vi "Logging Write.vi"(3 "error in (no error)":errorcluster, 5 "LoggingDevRef":T1) -> (0 "error out":errorcluster, 1 "Count":u32, 2 "LoggingDevRef":T1)   [LabVIEW 2012, in "femtoRoboLib.lvlib"]
doc: "Actually write unsaved log changes to to specified Logging reference. To prevent data loss, Flushing occasionally is recommended. Returns the number of changes written."
uses:
  femtoRoboLib.lvlib
  Controls/LoggingDevRef.ctl
  Controls/Logging Cache - Mode.ctl
  Controls/Log Entry - Written Block.ctl
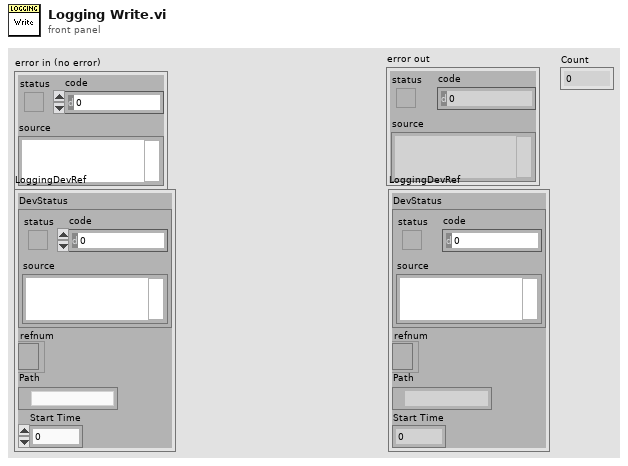
[diagram p1: front panel]
types:
  T1 = typedef "femtoRoboLib.lvlib/LoggingDevRef.ctl" = cluster{"DevStatus":errorcluster, "refnum":refnum<file>, "Path":path, "Start Time":u32}
  T2 = typedef "Log Entry - Written Block.ctl" = cluster{"ID":u32, "Value":string, "Type":enum16{"Boolean", "Numeric", "String", "Boolean Array", "Numeric Array", "String Array"}}
  T3 = typedef "Logging Cache - Mode.ctl" = enum16{"Set", "Get All", "Get Unsaved", "Get Unsaved and Clear", "Get New", "Get New and Clear"}
  T4 = typedef "femtoRoboLib.lvlib/Log Entry - Converted.ctl" = cluster{"Name":string, "Type":enum16{"Boolean", "Numeric", "String", "Boolean Array", "Numeric Array", "String Array"}, "Value":string, "ID":u32}
  T5 = enum16{"Boolean", "Numeric", "String", "Boolean Array", "Numeric Array", "String Array"}
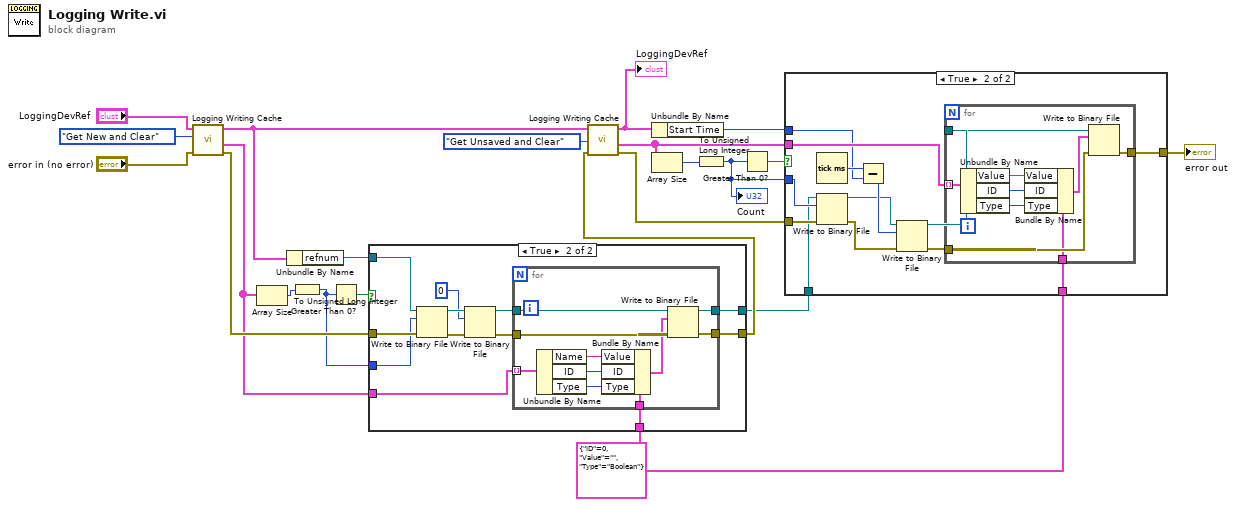
[diagram p0: block diagram]
diagram:
  w2 = T2 {"ID"=0, "Value"="", "Type"=enum."Boolean"} ("Log Entry - Written Block")
  n1 = call "Logging Writing Cache.vi"("error in (no error)"="error in (no error)", "Mode"=Logging_Cache_-_Mode."Get New and Clear", "LoggingDevRef"="LoggingDevRef") -> ("error out"=w6:errorcluster, "Out"=w4:T4[], "LoggingDevRef"=w8:T1)  [unwired: 2 in]
  n2 = Array Size(array=w4) -> (size(s)=w10:i32)
  n3 = Unbundle By Name(w8) -> ("refnum"=w7:refnum<file>)
  n4 = To Unsigned Long Integer(number=w10) -> (unsigned 32bit integer=w5:u32)
  n5 = Greater Than 0?(x=w5) -> (x > 0?=w9:bool)
  n6 = case shown="True" w9 {
    tunnel: w7 -> [w23 w36]
    tunnel: w6 -> [w24 w35]
    tunnel: w5 -> [_ w25]
    tunnel: w4 -> [_ w30]
    tunnel: [w24 w29] -> w3
    tunnel: w2 -> [_ w28]
    tunnel: [w23 w27] -> w1
    frame False {
    }
    frame True {
      n7 = Write to Binary File(file (use dialog)=w36, data=w25, error in=w35) -> (refnum out=w33:refnum<file>, error out=w34:errorcluster)  [unwired: 3 in, 1 out]
      n8 = Write to Binary File(file (use dialog)=w33, data=u32 0, error in=w34) -> (refnum out=w32:refnum<file>, error out=w31:errorcluster)  [unwired: 3 in, 1 out]
      n9 = for {
        tunnel: [w46] -> w29
        tunnel: w32 -> [w45]
        tunnel: w31 -> [w44]
        tunnel: w30 -> [w42] mode=indexing
        tunnel: w28 -> [w41]
        tunnel: [w37] -> w27
        n10 = Unbundle By Name(w42) -> ("Name"=w39:string, "ID"=w43:u32, "Type"=w38:T5)
        n11 = Bundle By Name(cluster=w41, "Value"=w39, "ID"=w43, "Type"=w38) -> (w40:T2)
        n12 = Write to Binary File(file (use dialog)=w45, data=w40, error in=w44) -> (refnum out=w37:refnum<file>, error out=w46:errorcluster)  [unwired: 3 in, 1 out]
      }
    }
  }
  n13 = call "Logging Writing Cache.vi"("error in (no error)"=w3, "Mode"=Logging_Cache_-_Mode."Get Unsaved and Clear", "LoggingDevRef"=w8) -> ("error out"=w20:errorcluster, "Out"=w19:T4[], "LoggingDevRef"=w21:T1)  [unwired: 2 in]
  "LoggingDevRef" <- w21
  n14 = Unbundle By Name(w21) -> ("Start Time"=w15:u32)
  n15 = Array Size(array=w19) -> (size(s)=w18:i32)
  n16 = To Unsigned Long Integer(number=w18) -> (unsigned 32bit integer=w16:u32)
  "Count" <- w16
  n17 = Greater Than 0?(x=w16) -> (x > 0?=w17:bool)
  n18 = case shown="True" w17 {
    tunnel: [w47 w60] -> w22
    tunnel: w20 -> [w47 w52]
    tunnel: w19 -> [_ w59]
    tunnel: w16 -> [_ w58]
    tunnel: w15 -> [_ w55]
    tunnel: w2 -> [_ w49]
    tunnel: w1 -> [_ w48]
    frame False {
    }
    frame True {
      n19 = Tick Count (ms)() -> (millisecond timer value=w56:u32)
      n20 = Write to Binary File(file (use dialog)=w48, data=w58, error in=w52) -> (refnum out=w53:refnum<file>, error out=w51:errorcluster)  [unwired: 3 in, 1 out]
      n21 = Subtract(x=w56, y=w55) -> (x-y=w57:u32)
      n22 = Write to Binary File(file (use dialog)=w53, data=w57, error in=w51) -> (refnum out=w54:refnum<file>, error out=w50:errorcluster)  [unwired: 3 in, 1 out]
      n23 = for {
        tunnel: w54 -> [w69]
        tunnel: w59 -> [w62] mode=indexing
        tunnel: w50 -> [w68]
        tunnel: [w67] -> w60
        tunnel: w49 -> [w63]
        n24 = Unbundle By Name(w62) -> ("Value"=w65:string, "ID"=w66:u32, "Type"=w61:T5)
        n25 = Bundle By Name(cluster=w63, "Value"=w65, "ID"=w66, "Type"=w61) -> (w64:T2)
        n26 = Write to Binary File(file (use dialog)=w69, data=w64, error in=w68) -> (error out=w67:errorcluster)  [unwired: 3 in, 2 out]
      }
    }
  }
  "error out" <- w22
